vi "Timer FGV.vi"(9 "타겟 시간 (s)":dbl, 11 "타이머 명령":T1) -> (1 "경과 시간":dbl, 2 "완료?":bool)   [LabVIEW 2010]
doc: "이 VI는 시작 명령이 VI에 전달된 후에 경과된 시간을 추적하는 기능적인 글로벌 변수입니다."
uses:
  TimerCommands.ctl
panel:
  # "입력"
  # "출력"
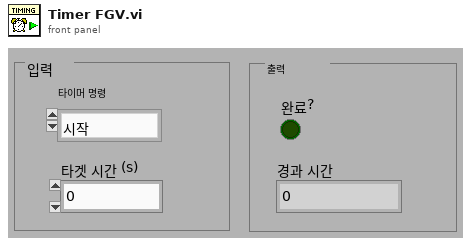
[diagram p1: front panel]
types:
  T1 = typedef "TimerCommands.ctl" = enum16{"시작", "시간 확인"}
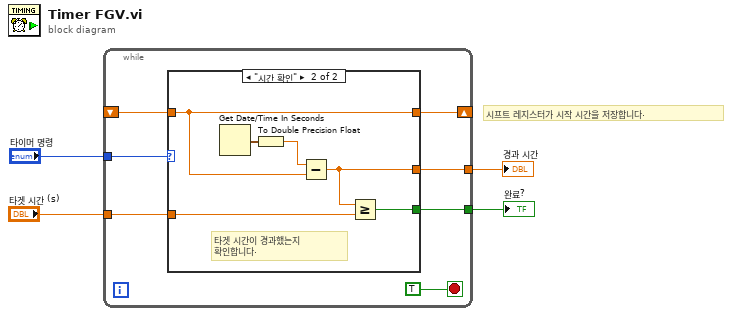
[diagram p0: block diagram]
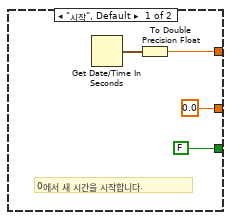
[diagram p2: hidden frame]
diagram:
  # "시프트 레지스터가 시작 시간을 저장합니다."
  n1 = while {
    tunnel: "타이머 명령" -> [w11]
    shift-right: [w10] -> _
    shift-left: _ -> [w9]
    tunnel: [w8] -> w3
    tunnel: [w7] -> w2
    tunnel: "타겟 시간 (s)" -> [w6]
    stop <- TRUE stop-if-true
    n2 = case shown="\"시간 확인\"" w11 {
      tunnel: [w14 w19] -> w10
      tunnel: w9 -> [_ w19]
      tunnel: [0.0 ("double precision float") w18] -> w8
      tunnel: [FALSE w17] -> w7
      tunnel: w6 -> [_ w16]
      frame "시작", Default {
        # "0에서 새 시간을 시작합니다."
        n3 = Get Date/Time In Seconds() -> (seconds since 1Jan1904=w15:timestamp)
        n4 = To Double Precision Float(number=w15) -> (double precision float=w14:dbl)
      }
      frame "시간 확인" {
        # "타겟 시간이 경과했는지 \n확인합니다."
        n5 = Get Date/Time In Seconds() -> (seconds since 1Jan1904=w21:timestamp)
        n6 = To Double Precision Float(number=w21) -> (double precision float=w20:dbl)
        n7 = Subtract(x=w20, y=w19) -> (x-y=w18:dbl)
        n8 = Greater Or Equal?(x=w18, y=w16) -> (x >= y?=w17:bool)
      }
    }
  }
  "경과 시간" <- w3
  "완료?" <- w2
